vi "NTCP Socket.vi"() -> ()   [LabVIEW 2013]
uses:
  NTCP library/NTCP Connection States.ctl
  NTCP library/NTCP Commands.ctl
  NTCP library/NTCP Log Msg.ctl
  lib/Launcher/NoPanelAppTypes.ctl
  lib/Launcher/Launcher Actions.ctl
  lib/Apps/App Parameters Actions.ctl
  lib/Data Access Objects/Metadata/LBCB Number.ctl
  lib/MixedMode/Messages/Target.ctl
  lib/NTCP Client/NTCP 2 MM Message.ctl
  lib/NTCP Client/NTCP Msg Types.ctl
  lib/Apps/Yes No Button.ctl
  lib/NTCP Client/MM 2 NTCP Message.ctl
  lib/Data Access Objects/Metadata/Persistant DAO Actions.ctl
  lib/Data Access Objects/Metadata/DAO Actions.ctl
panel:
  out "timeout":i32=500
  in  "error in (no error)":errorcluster
  out "stopped":bool
  out "NTCP Connection State":T1=enum."Listen"
  out "Remote ID":refnum<k5>
  out "Transaction ID":string
  out "Response":string
  out "Response Time Stamp":string
  out "Connected":bool
  out "Client IP":string
  out "Incoming Command":string
  out "Command Time Stamp":string
  out "Port":u16=6342
  out "Logfile":path=path "C:/temp/ntcp-0719.txt"
  out "Command Received":i32
  out "Host IP":string="http://cee-zzim.cee.uiuc.edu"
  # "NTCP Communication Socket"
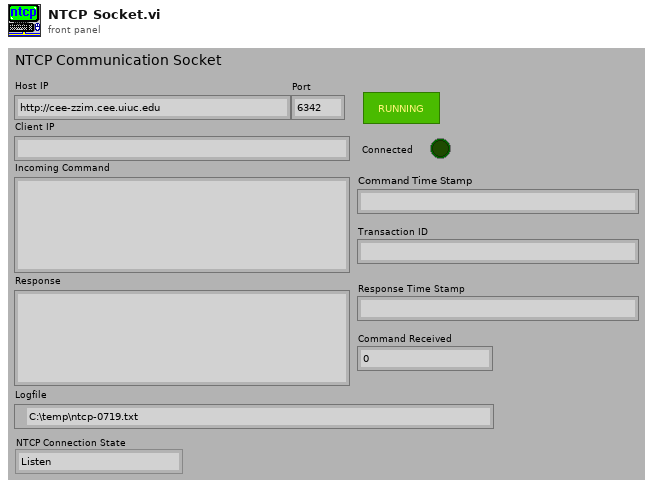
[diagram p1: front panel]
types:
  T1 = typedef "NTCP Connection States.ctl" = enum16{"Init", "Listen", "Read", "Start Local Shutdown", "Close", "Send Proposed", "Wait for Propose Response", "Reply Close Session", "Send Control Point", "Reply Unknown", "Reply Cancel", "Reply Set Parameter", "Reply Get Parameter", "Send Execute Request", "Wait for Execute Response", "Reply Open Session"}
  T2 = typedef "MM 2 NTCP Message.ctl" = cluster{"NTCP commands":T3, "Transaction ID":string, "Control Point":string, "Accepted":T4}
  T3 = typedef "NTCP Commands.ctl" = enum16{"propose", "execute", "cancel", "set-parameter", "get-parameter", "open-session", "close-session", "get-control-point", "Unknown", "stop"}
  T4 = typedef "Yes No Button.ctl" = bool
  T5 = typedef "NTCP 2 MM Message.ctl" = cluster{"NTCP commands":T3, "Transaction ID":string, "Control Point":string, "Targets":T6[]}
  T6 = typedef "Target.ctl" = cluster{"LBCB Number":T7, "DOF Vectors":enum16{" ", "Dx", "Dy", "Dz", "Rx", "Ry", "Rz", "Fx", "Fy", "Fz", "Mx", "My", "Mz"}, "Amount":dbl}
  T7 = typedef "LBCB Number.ctl" = enum16{"LBCB1", "LBCB2"}
  T8 = typedef "DAO Actions.ctl" = enum16{"Init", "Get", "Set"}
  T9 = typedef "Persistant DAO Actions.ctl" = enum16{"Init", "Get", "Set", "Load", "Save"}
  T10 = typedef "Network Parameters.ctl" = cluster{"Port Number":u16, "Notification Name":string, "Wait For Notification Timeout":i32}
  T11 = typedef "App Parameters Actions.ctl" = enum16{"Init", "Get", "Set"}
  T12 = typedef "NTCP Log Msg.ctl" = enum16{"None", "Command", "Response"}
  T13 = enum16{"Standard", "Buffered", "CRLF", "Immediate"}
  T14 = typedef "NTCP Msg Types.ctl" = enum16{"Control Point", "Step Done", "Propose Accepted", "Propose Not Accepted", "Propose Declined", "Propose Response", "Execute Done", "Offsets", "Initial Position"}
  T15 = typedef "App Parameters.ctl" = cluster{"Monitor Loop":T16, "Ramp Time":T16, "Log Loop":T16, "TCP to DAQ":T16, "Logging Directory":path, "Log File Size (MBytes)":i64, "Volt Logging Loop":T16, "2 LBCB Archiving Mode":bool, "Fake":bool}
  T16 = typedef "Timing Parameters.ctl" = cluster{"Interval":dbl, "Rate ":dbl}
  T17 = typedef "NTCP Message.ctl" = cluster{"NTCP commands":T3, "Transaction ID":string, "Control Point":string, "Payloads":T18[]}
  T18 = typedef "Payload.ctl" = cluster{"Content":string, "Control Point Suffix":T19}
  T19 = typedef "Control Point Suffix.ctl" = enum16{"LBCB1", "LBCB2", "ExternalSensors"}
  T20 = typedef "Launcher Actions.ctl" = enum16{"Launch", "Stop All", "Stop", "Kill", "Running?", "Init"}
  T21 = typedef "NoPanelAppTypes.ctl" = enum16{"NTCP Socket", "Data Archiving", "DAQ Link", "Control Loops", "Cmd Disp Diffs", "LBCB Data", "Limits", "Mixed Mode Widget", "Offsets", "Debug"}
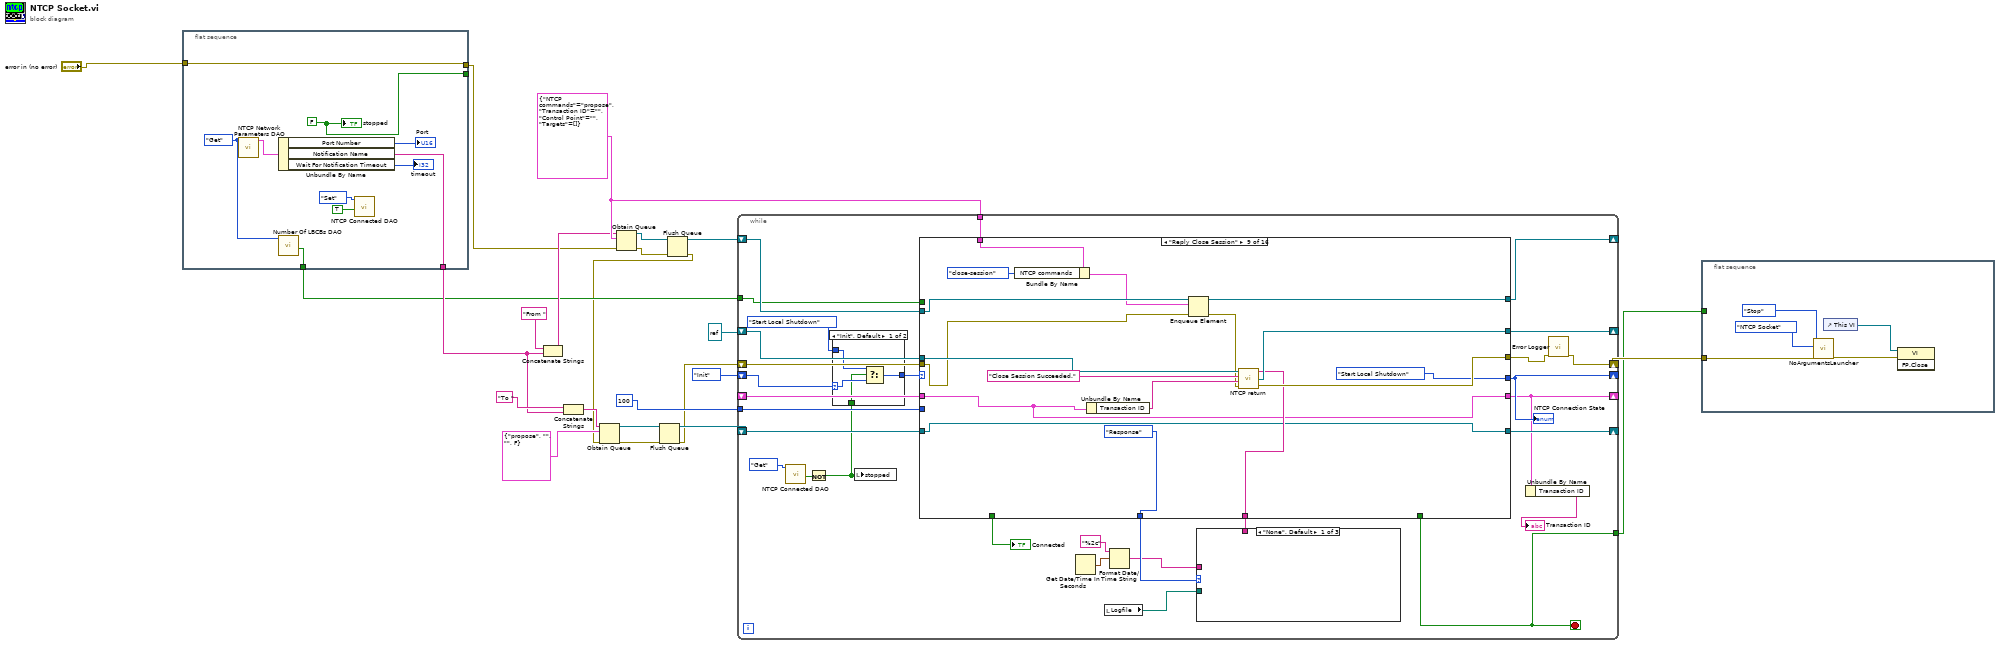
[diagram p0: block diagram]
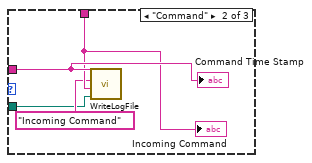
[diagram p3: hidden frame]
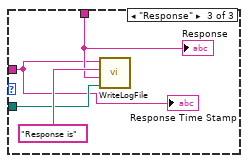
[diagram p4: hidden frame]
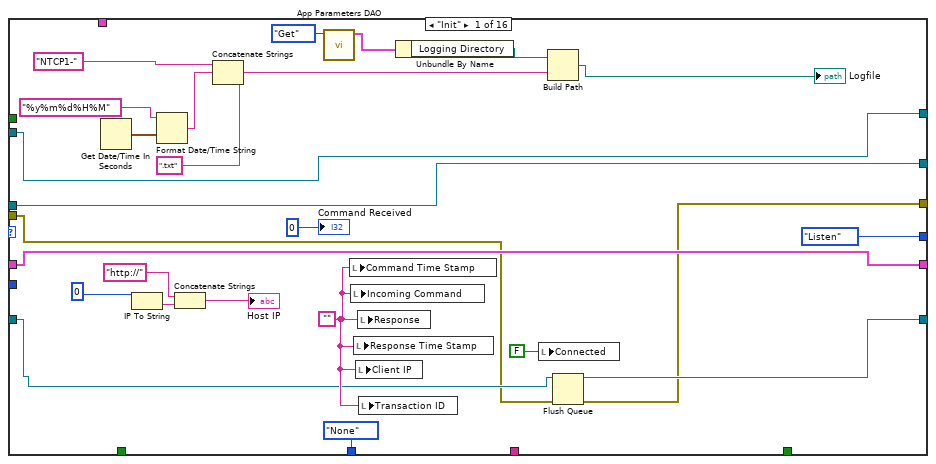
[diagram p5: hidden frame]
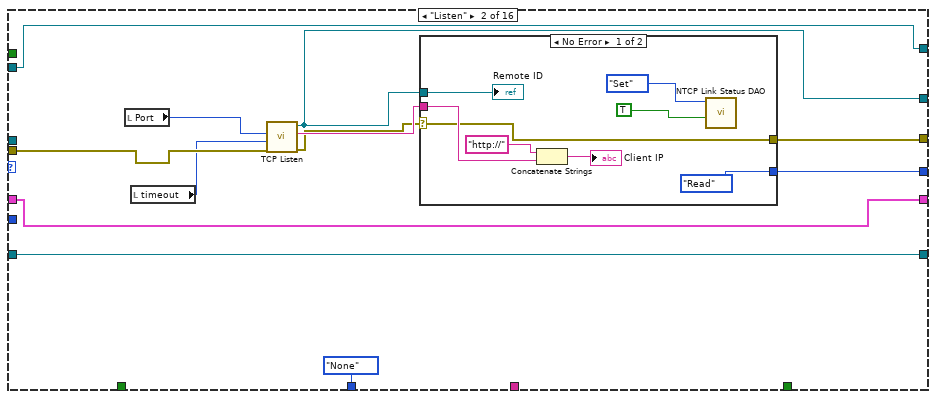
[diagram p6: hidden frame]
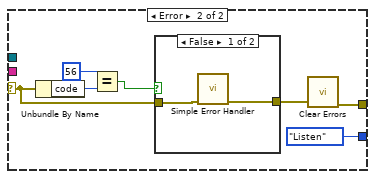
[diagram p7: hidden frame]
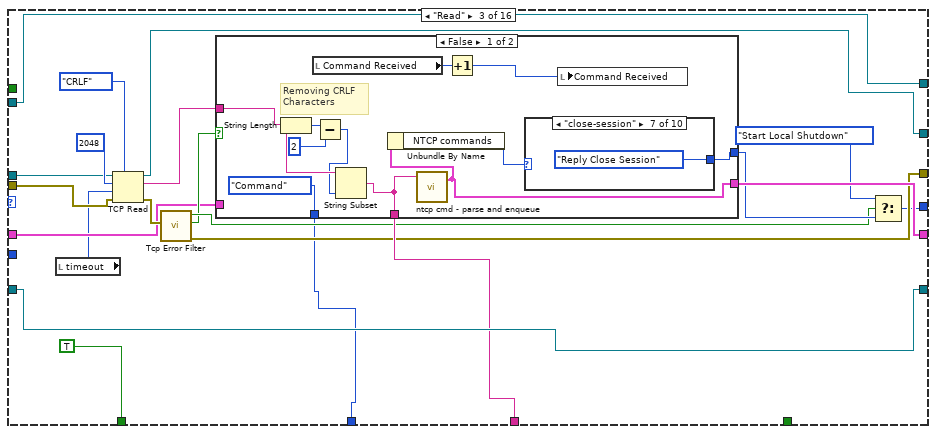
[diagram p9: hidden frame]
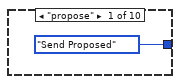
[diagram p10: hidden frame]
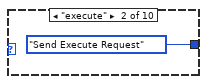
[diagram p11: hidden frame]
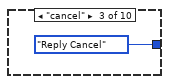
[diagram p12: hidden frame]
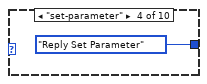
[diagram p13: hidden frame]
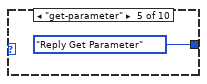
[diagram p14: hidden frame]
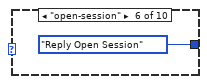
[diagram p15: hidden frame]
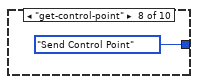
[diagram p16: hidden frame]
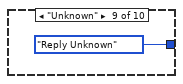
[diagram p17: hidden frame]
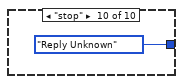
[diagram p18: hidden frame]
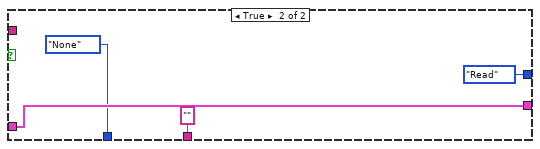
[diagram p19: hidden frame]
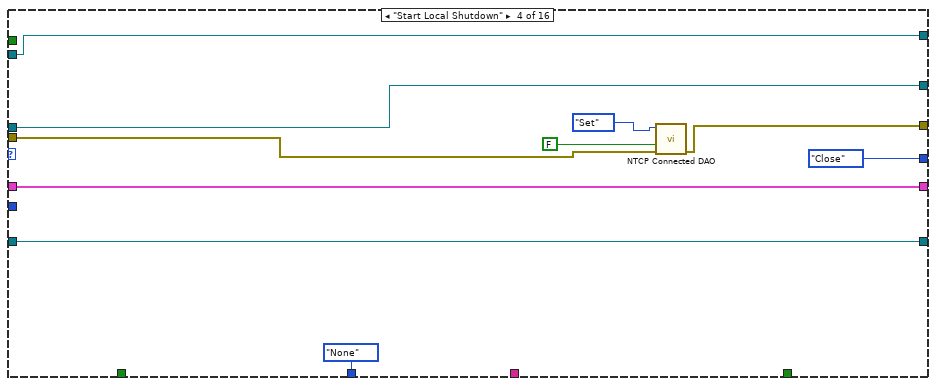
[diagram p20: hidden frame]
diagram:
  w17 = T5 {"NTCP commands"=enum."propose", "Transaction ID"="", "Control Point"="", "Targets"=[]} ("NTCP Message")
  n1 = flat-sequence {
    tunnel: [w27] -> w8
    tunnel: [w30] -> w11
    tunnel: [w28] -> w10
    tunnel: "error in (no error)" -> [w27]
    tunnel: [w26] -> _
    frame #0 {
      w29 = Persistant_DAO_Actions."Get" ("Persistent DAO Actions")
      w26 = FALSE ("running")
      n2 = call "NTCP Network Parameters DAO.vi"("Persistent DAO Actions"=w29) -> ("Network Parameters Out"=w33:T10)  [unwired: 8 in, 2 out]
      n3 = Unbundle By Name(w33) -> ("Port Number"=→"Port":u16, "Notification Name"=w30:string, "Wait For Notification Timeout"=→"timeout":i32)
      n4 = call "Number Of LBCBs DAO.vi"("Actions"=w29) -> ("Rigid Connection Out"=w28:bool)  [unwired: 7 in, 3 out]
      n5 = call "NTCP Connected DAO.vi"("NTCP Connected In"=TRUE, "DAO Actions"=DAO_Actions."Set") -> ()  [unwired: 8 in, 2 out]
      "stopped" <- w26
    }
  }
  n6 = Concatenate Strings("From " ("name (unnamed)"), w11) -> (w14:string)
  n7 = Concatenate Strings("To " ("name (unnamed)"), w11) -> (w13:string)
  n8 = Obtain Queue(name (unnamed)=w14, element data type=w17, error in (no error)=w8) -> (queue out=w22:refnum<queue>, error out=w3:errorcluster)  [unwired: 2 in, 1 out]
  n9 = Flush Queue(queue=w22, error in (no error)=w3) -> (queue out=w4:refnum<queue>, error out=w2:errorcluster)  [unwired: 1 out]
  n10 = Obtain Queue(name (unnamed)=w13, element data type=T2 {"NTCP commands"=enum."propose", "Transaction ID"="", "Control Point"="", "Accepted"=FALSE} ("NTCP Message"), error in (no error)=w2) -> (queue out=w21:refnum<queue>, error out=w6:errorcluster)  [unwired: 2 in, 1 out]
  n11 = Flush Queue(queue=w21, error in (no error)=w6) -> (queue out=w7:refnum<queue>, error out=w5:errorcluster)  [unwired: 1 out]
  n12 = while {
    shift-right: [w63] -> _
    shift-left: refnum<k5> refnum ("connection ID out") -> [w60]
    shift-right: [w44] -> w18
    shift-left: w5 -> [w59]
    shift-right: [w47] -> _
    shift-left: _ -> [w61]
    shift-right: [w62] -> _
    shift-left: NTCP_Connection_States."Init" ("NTCP Connection State") -> [w40]
    shift-right: [w57] -> _
    shift-left: w4 -> [w58]
    tunnel: 100 ("timeout in ms (-1)") -> [w55]
    shift-right: [w54] -> _
    shift-left: w7 -> [w56]
    tunnel: [w42] -> w1
    tunnel: w17 -> [w41]
    tunnel: w10 -> [w37]
    stop <- w42 stop-if-true
    n13 = call "NTCP Connected DAO.vi"("DAO Actions"=DAO_Actions."Get") -> ("NTCP Connected Out"=w35:bool)  [unwired: 9 in, 1 out]
    n14 = Not(x=w35) -> (.not. x?=w34:bool)
    n15 = case shown="\"Init\", Default" w40 {
      selector: w40 -> [w66 w68]
      tunnel: NTCP_Connection_States."Start Local Shutdown" ("f") -> [w67 _]
      tunnel: [w65 w68] -> w38
      tunnel: w34 -> [w64 _]
      frame "Init", Default {
        n16 = Select(t=w67, s=w64, f=w66) -> (s? t:f=w65:T1)
      }
      frame "Close" {
      }
    }
    n17 = local write "stopped"(w34) -> ()
    n18 = case shown="\"Reply Close Session\"" w38 {
      tunnel: [w91 w112 w150 w183 w204 w220 w233 w264 w301 w307 w332 w358 w371 w384 w395 w412] -> w63
      tunnel: [NTCP_Connection_States."Listen" ("NTCP Connection State") w104 w140 NTCP_Connection_States."Close" ("NTCP Connection State") NTCP_Connection_States."Close" ("NTCP Connection State") NTCP_Connection_States."Wait for Propose Response" ("NTCP Connection State") w228 w258 NTCP_Connection_States."Start Local Shutdown" ("NTCP Connection State") NTCP_Connection_States."Read" ("NTCP Connection State") NTCP_Connection_States."Read" ("NTCP Connection State") NTCP_Connection_States."Read" ("NTCP Connection State") NTCP_Connection_States."Read" ("NTCP Connection State") NTCP_Connection_States."Read" ("NTCP Connection State") NTCP_Connection_States."Wait for Execute Response" ("NTCP Connection State") NTCP_Connection_States."Read" ("NTCP Connection State")] -> w62
      tunnel: [w90 w111 w152 w187 w192 w214 w226 w259 w294 w317 w342 w351 w364 w377 w391 w405] -> w47
      tunnel: w61 -> [w90 w111 w136 w187 w192 w214 w226 w259 w294 w317 w342 w351 w364 w377 w391 w405]
      tunnel: w60 -> [w91 _ w151 w183 w205 w220 w234 w265 w302 w308 w333 w359 w372 w385 w395 w413]
      tunnel: w59 -> [w77 w110 w149 w181 w206 w216 w232 w263 w290 w310 w335 w357 w370 w383 w398 w411]
      tunnel: [w84 w105 w144 w180 w195 w222 w231 w262 w300 w309 w334 w356 w369 w382 w397 w410] -> w45
      tunnel: [_ _ _ _ TRUE _ _ _ _ _ _ _ _ _ _ _] -> w42
      tunnel: w58 -> [w78 w109 w148 w184 w197 w224 w227 w257 w292 w318 w343 w349 w362 w375 w400 w403]
      tunnel: [w78 w109 w148 w184 w196 w223 w227 w257 w291 w318 w343 w349 w362 w375 w399 w403] -> w57
      tunnel: w56 -> [w86 w108 w147 w185 w203 w219 w239 w270 w296 w320 w345 w352 w365 w378 w394 w406]
      tunnel: w55 -> [_ _ _ _ _ _ w238 w269 _ _ _ _ _ _ _ _]
      tunnel: [w85 w108 w147 w185 w203 w219 w237 w268 w296 w320 w345 w352 w365 w378 w394 w406] -> w54
      tunnel: [NTCP_Log_Msg."None" ("Log Msg") NTCP_Log_Msg."None" ("Log Msg") w135 NTCP_Log_Msg."None" ("Log Msg") NTCP_Log_Msg."None" ("Log Msg") NTCP_Log_Msg."None" ("Log Msg") w229 w260 NTCP_Log_Msg."Response" ("Log Msg") NTCP_Log_Msg."Response" ("Log Msg") NTCP_Log_Msg."Response" ("Log Msg") NTCP_Log_Msg."Response" ("Log Msg") NTCP_Log_Msg."Response" ("Log Msg") NTCP_Log_Msg."Response" ("Log Msg") NTCP_Log_Msg."None" ("Log Msg") NTCP_Log_Msg."Response" ("Log Msg")] -> w51
      tunnel: [_ _ w146 _ _ _ w230 w261 w299 w305 w330 w355 w368 w381 _ w409] -> w49
      tunnel: [_ _ TRUE _ _ TRUE TRUE TRUE _ TRUE TRUE TRUE TRUE TRUE TRUE TRUE] -> w43
      tunnel: w41 -> [_ _ _ _ w193 w212 _ _ w288 _ _ _ _ _ w392 _]
      tunnel: w37 -> [_ _ _ _ _ _ _ _ _ w303 w322 _ _ _ _ _]
      frame "Init" {
        w92 = ""
        n19 = Get Date/Time In Seconds() -> (seconds since 1Jan1904=w99:timestamp)
        n20 = IP To String(2:0) -> (0:w94:string)  [unwired: 1 out]
        n21 = Format Date/Time String(time format string (%c)="%y%m%d%H%M", seconds (now)=w99) -> (date/time string=w100:string)  [unwired: 1 out]
        n22 = Concatenate Strings("http://", w94) -> (→"Host IP":string)
        n23 = Concatenate Strings("NTCP1-", w100, ".txt") -> (w80:string)
        n24 = call "App Parameters DAO.vi"("Actions"=App_Parameters_Actions."Get" ("App Parameter Actions")) -> ("Application Timing and Logging Out"=w82:T15)  [unwired: 3 in, 7 out]
        n25 = local write "Command Time Stamp"(w92) -> ()
        n26 = local write "Incoming Command"(w92) -> ()
        n27 = local write "Response Time Stamp"(w92) -> ()
        n28 = local write "Client IP"(w92) -> ()
        n29 = local write "Response"(w92) -> ()
        n30 = local write "Transaction ID"(w92) -> ()
        n31 = Unbundle By Name(w82) -> ("Logging Directory"=w81:path)
        n32 = local write "Connected"(FALSE) -> ()
        n33 = Build Path(base path=w81, name or relative path=w80) -> (appended path=→"Logfile":path)
        n34 = Flush Queue(queue=w86, error in (no error)=w77) -> (queue out=w85:refnum<queue>, error out=w84:errorcluster)  [unwired: 1 out]
        "Command Received" <- 0
      }
      frame "Listen" {
        n35 = local read "Port"() -> (w114:u16)
        n36 = local read "timeout"() -> (w103:i32)
        n37 = call <vilib>:"TCP Listen.vi"("error in (no error)"=w110, "timeout ms (wait forever: -1)"=w103, "port"=w114) -> ("error out"=w106:errorcluster, "remote address"=w113:string, "connection ID"=w112:refnum<k5>)  [unwired: 1 in, 5 out]
        n38 = case shown="No Error" w106 {
          selector: w106 -> [w118 w126]
          tunnel: w113 -> [w121 _]
          tunnel: w112 -> [w119 _]
          tunnel: [w118 w124] -> w105
          tunnel: [NTCP_Connection_States."Read" ("NTCP Connection State") NTCP_Connection_States."Listen" ("NTCP Connection State")] -> w104
          frame No Error {
            n39 = Concatenate Strings("http://", w121) -> (→"Client IP":string)
            n40 = call "NTCP Link Status DAO.vi"("NTCP Link In"=TRUE ("Status\nSetting"), "DAO Actions"=DAO_Actions."Set") -> ()  [unwired: 8 in, 2 out]
            "Remote ID" <- w119
          }
          frame Error {
            n41 = Unbundle By Name(w126) -> ("code"=w129:i32)
            n42 = Equal?(x=56, y=w129) -> (x = y?=w127:bool)
            n43 = case shown="False" w127 {
              tunnel: w126 -> [w131 w132]
              tunnel: [w130 w132] -> w125
              frame False {
                n44 = call <vilib>:"Simple Error Handler.vi"("error in (no error)"=w131) -> ("error out"=w130:errorcluster)  [unwired: 1 in, 7 out]
              }
              frame True {
              }
            }
            n45 = call <vilib>:"Clear Errors.vi"("error in (no error)"=w125) -> ("error out"=w124:errorcluster)  [unwired: 6 out]
          }
        }
      }
      frame "Read" {
        n46 = local read "timeout"() -> (w133:i32)
        n47 = TCP Read(connection ID=w151, bytes to read=2048, error in (no error)=w149, 7:T13."CRLF" ("mode (standard)"), 9:w133) -> (connection ID out=w150:refnum<k5>, data out=w138:string, error out=w145:errorcluster)
        n48 = call "Tcp Error Filter.vi"("error in (no error)"=w145) -> ("error out"=w144:errorcluster, "Timed Out"=w137:bool, "Lost"=w141:bool)  [unwired: 8 out]
        n49 = case shown="False" w137 {
          tunnel: [w164 w177] -> w152
          tunnel: [w163 "" ("data out")] -> w146
          tunnel: [w162 NTCP_Connection_States."Read" ("NTCP Connection State")] -> w143
          tunnel: w138 -> [w161 _]
          tunnel: w136 -> [_ w177]
          tunnel: [NTCP_Log_Msg."Command" ("Log Msg") NTCP_Log_Msg."None" ("Log Msg")] -> w135
          frame False {
            # "Removing CRLF\nCharacters"
            n50 = String Length(string=w161) -> (length=w160:i32)
            n51 = local read "Command Received"() -> (w157:i32)
            n52 = Subtract(x=w160, y=2) -> (x-y=w158:i32)
            n53 = String Subset(string=w161, length (rest)=w158) -> (substring=w163:string)  [unwired: 1 out]
            n54 = call "ntcp cmd - parse and enqueue.vi"("Command from NTCP"=w163) -> ("message"=w164:T17)  [unwired: 3 out]
            n55 = Unbundle By Name(w164) -> ("NTCP commands"=w155:T3)
            n56 = Increment(x=w157) -> (x+1=w156:i32)
            n57 = case shown="\"close-session\"" w155 {
              tunnel: [NTCP_Connection_States."Send Proposed" ("NTCP Connection State") NTCP_Connection_States."Send Execute Request" ("NTCP Connection State") NTCP_Connection_States."Reply Cancel" ("NTCP Connection State") NTCP_Connection_States."Reply Set Parameter" ("NTCP Connection State") NTCP_Connection_States."Reply Get Parameter" ("NTCP Connection State") NTCP_Connection_States."Reply Open Session" ("NTCP Connection State") NTCP_Connection_States."Reply Close Session" ("NTCP Connection State") NTCP_Connection_States."Send Control Point" ("NTCP Connection State") NTCP_Connection_States."Reply Unknown" ("NTCP Connection State") NTCP_Connection_States."Reply Unknown" ("NTCP Connection State")] -> w162
              frame "propose" {
              }
              frame "execute" {
              }
              frame "cancel" {
              }
              frame "set-parameter" {
              }
              frame "get-parameter" {
              }
              frame "open-session" {
              }
              frame "close-session" {
              }
              frame "get-control-point" {
              }
              frame "Unknown" {
              }
              frame "stop" {
              }
            }
            n58 = local write "Command Received"(w156) -> ()
          }
          frame True {
          }
        }
        n59 = Select(t=NTCP_Connection_States."Start Local Shutdown", s=w141, f=w143) -> (s? t:f=w140:T1)
      }
      frame "Start Local Shutdown" {
        n60 = call "NTCP Connected DAO.vi"("error in (no error)"=w181, "NTCP Connected In"=FALSE ("NTCP Link In"), "DAO Actions"=DAO_Actions."Set") -> ("error out"=w180:errorcluster)  [unwired: 7 in, 1 out]
      }
      frame "Close" {
        n61 = Unbundle By Name(w192) -> ("NTCP commands"=w191:T3)
        n62 = TCP Close Connection(connection ID=w205, error in (no error)=w206) -> (connection ID out=w204:refnum<k5>, error out=w207:errorcluster)  [unwired: 1 out]
        n63 = call "NTCP Link Status DAO.vi"("NTCP Link In"=FALSE ("Status\nSetting"), "DAO Actions"=DAO_Actions."Set") -> ()  [unwired: 8 in, 2 out]
        n64 = call <vilib>:"Clear Errors.vi"("error in (no error)"=w207) -> ("error out"=w190:errorcluster)  [unwired: 6 out]
        n65 = Bundle By Name(cluster=w193, "NTCP commands"=w191) -> (w198:T5)
        n66 = Enqueue Element(queue=w197, element=w198, error in (no error)=w190) -> (queue out=w196:refnum<queue>, error out=w194:errorcluster)  [unwired: 2 out]
        n67 = Merge Errors(w194, w190) -> (w195:errorcluster)
      }
      frame "Send Proposed" {
        n68 = Unbundle By Name(w214) -> ("NTCP commands"=w210:T3, "Payloads"=w213:T18[], "Transaction ID"=w208:string)
        n69 = call "NTCP Propose 2 Targets.vi"("error in"=w216, "Payload"=w213) -> ("error out"=w215:errorcluster, "Step Out"=w211:T6[])
        n70 = Bundle By Name(cluster=w212, "NTCP commands"=w210, "Targets"=w211, "Transaction ID"=w208) -> (w209:T5)
        n71 = Enqueue Element(queue=w224, element=w209, error in (no error)=w215) -> (queue out=w223:refnum<queue>, error out=w222:errorcluster)  [unwired: 2 out]
      }
      frame "Wait for Propose Response" {
        n72 = Dequeue Element(queue=w239, timeout in ms (-1)=w238) -> (queue out=w237:refnum<queue>, element=w235:T2, timed out?=w236:bool)  [unwired: 1 in, 1 out]
        n73 = case shown="False" w236 {
          tunnel: w235 -> [w244 _]
          tunnel: w234 -> [w251 w255]
          tunnel: [w250 w255] -> w233
          tunnel: w232 -> [w249 w254]
          tunnel: [w248 w254] -> w231
          tunnel: [w247 _] -> w230
          tunnel: [NTCP_Log_Msg."Response" ("Log Msg") NTCP_Log_Msg."None" ("Log Msg")] -> w229
          tunnel: [NTCP_Connection_States."Read" ("NTCP Connection State") NTCP_Connection_States."Wait for Propose Response" ("NTCP Connection State")] -> w228
          tunnel: w226 -> [w242 _]
          frame False {
            n74 = Unbundle By Name(w244) -> ("Accepted"=w243:T4)
            n75 = Unbundle By Name(w242) -> ("Transaction ID"=w241:string)
            n76 = call "NTCP return.vi"("NTCP Server"=w251, "Message Body"="Accepted", "Transaction ID"=w241, "NTCP return error"=w249, "Response OK"=w243) -> ("Response string"=w247:string, "connection ID out"=w250:refnum<k5>, "error out"=w248:errorcluster)
          }
          frame True {
          }
        }
      }
      frame "Wait for Execute Response" {
        n77 = Dequeue Element(queue=w270, timeout in ms (-1)=w269) -> (queue out=w268:refnum<queue>, element=w266:T2, timed out?=w267:bool)  [unwired: 1 in, 1 out]
        n78 = case shown="False" w267 {
          tunnel: w266 -> [w273 _]
          tunnel: w265 -> [w281 w285]
          tunnel: [w280 w285] -> w264
          tunnel: w263 -> [w278 w284]
          tunnel: [w277 w284] -> w262
          tunnel: [w276 _] -> w261
          tunnel: [NTCP_Log_Msg."Response" ("Log Msg") NTCP_Log_Msg."None" ("Log Msg")] -> w260
          tunnel: [NTCP_Connection_States."Read" ("NTCP Connection State") NTCP_Connection_States."Wait for Propose Response" ("NTCP Connection State")] -> w258
          frame False {
            n79 = Unbundle By Name(w273) -> ("Accepted"=w272:T4, "Transaction ID"=w279:string)
            n80 = call "NTCP return.vi"("NTCP Server"=w281, "Message Body"="Execute is done", "Transaction ID"=w279, "NTCP return error"=w278, "Response OK"=w272) -> ("Response string"=w276:string, "connection ID out"=w280:refnum<k5>, "error out"=w277:errorcluster)
          }
          frame True {
          }
        }
      }
      frame "Reply Close Session" {
        n81 = Bundle By Name(cluster=w288, "NTCP commands"=NTCP_Commands."close-session") -> (w287:T5)
        n82 = Unbundle By Name(w294) -> ("Transaction ID"=w297:string)
        n83 = Enqueue Element(queue=w292, element=w287, error in (no error)=w290) -> (queue out=w291:refnum<queue>, error out=w289:errorcluster)  [unwired: 1 in, 1 out]
        n84 = call "NTCP return.vi"("NTCP Server"=w302, "Message Body"="Close Session Succeeded." ("source"), "Transaction ID"=w297, "NTCP return error"=w289) -> ("Response string"=w299:string, "connection ID out"=w301:refnum<k5>, "error out"=w300:errorcluster)  [unwired: 1 in]
      }
      frame "Send Control Point" {
        n85 = Unbundle By Name(w317) -> ("Transaction ID"=w316:string, "Control Point"=w315:string, "Payloads"=w313:T18[])
        n86 = Index Array(array=w313, index=0) -> (element=w312:T18)
        n87 = Unbundle By Name(w312) -> ("Control Point Suffix"=w311:T19)
        n88 = call "NTCP Send Msgs.vi"("Message Type"=NTCP_Msg_Types."Control Point", "NTCP Server In"=w308, "Combined"=w303, "Transaction ID"=w316, "Contol\nPoint\nSuffix"=w311, "ControlPoint name"=w315, "error in (no error)"=w310) -> ("Message"=w305:string, "NTCP Server Out"=w307:refnum<k5>, "error out"=w309:errorcluster)  [unwired: 3 in, 3 out]
      }
      frame "Reply Get Parameter" {
        n89 = Unbundle By Name(w342) -> ("Transaction ID"=w341:string, "Control Point"=w340:string, "Payloads"=w338:T18[])
        n90 = Index Array(array=w338, index=0) -> (element=w337:T18)
        n91 = Unbundle By Name(w337) -> ("Control Point Suffix"=w336:T19, "Content"=w327:string)
        n92 = Match Pattern(string=w327, regular expression="offsets") -> (offset past match=w325:i32)  [unwired: 1 in, 3 out]
        n93 = Greater Or Equal To 0?(x=w325) -> (x >= 0?=w324:bool)
        n94 = Select(t=NTCP_Msg_Types."Offsets" ("Message Type"), s=w324, f=NTCP_Msg_Types."Initial Position") -> (s? t:f=w328:T14)
        n95 = call "NTCP Send Msgs.vi"("Message Type"=w328, "NTCP Server In"=w333, "Combined"=w322, "Transaction ID"=w341, "Contol\nPoint\nSuffix"=w336, "ControlPoint name"=w340, "error in (no error)"=w335) -> ("Message"=w330:string, "NTCP Server Out"=w332:refnum<k5>, "error out"=w334:errorcluster)  [unwired: 3 in, 3 out]
      }
      frame "Reply Unknown" {
        n96 = Unbundle By Name(w351) -> ("Transaction ID"=w353:string)
        n97 = call "NTCP return.vi"("NTCP Server"=w359, "Message Body"="Unimplemented command", "Transaction ID"=w353, "NTCP return error"=w357) -> ("Response string"=w355:string, "connection ID out"=w358:refnum<k5>, "error out"=w356:errorcluster)  [unwired: 1 in]
      }
      frame "Reply Cancel" {
        n98 = Unbundle By Name(w364) -> ("Transaction ID"=w366:string)
        n99 = call "NTCP return.vi"("NTCP Server"=w372, "Message Body"="Cancel Ignored" ("source"), "Transaction ID"=w366, "NTCP return error"=w370) -> ("Response string"=w368:string, "connection ID out"=w371:refnum<k5>, "error out"=w369:errorcluster)  [unwired: 1 in]
      }
      frame "Reply Set Parameter" {
        n100 = Unbundle By Name(w377) -> ("Transaction ID"=w379:string)
        n101 = call "NTCP return.vi"("NTCP Server"=w385, "Message Body"="Command ignored. Carry on.", "Transaction ID"=w379, "NTCP return error"=w383) -> ("Response string"=w381:string, "connection ID out"=w384:refnum<k5>, "error out"=w382:errorcluster)  [unwired: 1 in]
      }
      frame "Send Execute Request" {
        n102 = Unbundle By Name(w391) -> ("NTCP commands"=w390:T3, "Transaction ID"=w389:string, "Control Point"=w388:string)
        n103 = Bundle By Name(cluster=w392, "NTCP commands"=w390, "Transaction ID"=w389, "Control Point"=w388) -> (w387:T5)
        n104 = Enqueue Element(queue=w400, element=w387, error in (no error)=w398) -> (queue out=w399:refnum<queue>, error out=w397:errorcluster)  [unwired: 2 out]
      }
      frame "Reply Open Session" {
        n105 = Unbundle By Name(w405) -> ("Transaction ID"=w407:string)
        n106 = call "NTCP return.vi"("NTCP Server"=w413, "Message Body"="Open Session Succeeded." ("source"), "Transaction ID"=w407, "NTCP return error"=w411) -> ("Response string"=w409:string, "connection ID out"=w412:refnum<k5>, "error out"=w410:errorcluster)  [unwired: 1 in]
      }
    }
    "NTCP Connection State" <- w62
    "Connected" <- w43
    n107 = Get Date/Time In Seconds() -> (seconds since 1Jan1904=w52:timestamp)
    n108 = local read "Logfile"() -> (w48:path)
    n109 = Format Date/Time String(time format string (%c)="%2c", seconds (now)=w52) -> (date/time string=w50:string)  [unwired: 1 out]
    n110 = case shown="\"None\", Default" w51 {
      tunnel: w50 -> [_ w72 w73]
      tunnel: w49 -> [_ w71 w74]
      tunnel: w48 -> [_ w69 w75]
      frame "None", Default {
      }
      frame "Command" {
        n111 = call "WriteLogFile.vi"("Logfile"=w69, "Message"=w71, "Caller"="Incoming Command", "Time"=w72) -> ()
        "Command Time Stamp" <- w72
        "Incoming Command" <- w71
      }
      frame "Response" {
        n112 = call "WriteLogFile.vi"("Logfile"=w75, "Message"=w74, "Caller"="Response is", "Time"=w73) -> ()
        "Response" <- w74
        "Response Time Stamp" <- w73
      }
    }
    n113 = Unbundle By Name(w47) -> ("Transaction ID"=→"Transaction ID":string)
    n114 = call "Error Logger.vi"("error in (no error)"=w45) -> ("error out"=w44:errorcluster)  [unwired: 1 in, 9 out]
  }
  n115 = flat-sequence {
    tunnel: w18 -> [w414]
    tunnel: w1 -> [_]
    frame #0 {
      n116 = call "NoArgumentsLauncher.vi"("error in (no error)"=w414, "Application"=NoPanelAppTypes."NTCP Socket", "Application Launcher Actions"=Launcher_Actions."Stop") -> ("error out"=w415:errorcluster)  [unwired: 8 out]
      n117 = control-ref of="This VI"() -> (w416:refnum<vi>)
      n118 = invoke class="VI" method="FP.Close"(reference=w416, error in=w415) -> ()  [unwired: 1 in, 3 out]
    }
  }
